vi "RFmxSpecAn CHP (Analysis Only) with Recommended Settings -Out of the Box.vi"() -> ()   [LabVIEW 2017]
doc: "This example illustrates how to use NI-RFmx in hardware agnostic mode to perform measurements on user provided IQ or Spectrum waveform. The example uses NI-RFSA driver API to acquire waveform from NI RF Signal Analyzer and perform an ACP measurement. The NI-RFSA acquisition settings are read from NI-RFmx session after Commit VI call. The NI-RFmx session is opened with Option String set as \"AnalysisOnly=1\"."
uses:
  <vilib>/Utility/error.llb/DialogType.ctl
  <instrlib>/niRFSA/niRFSA.llb/niRFSA Fetch IQ (1D Complex WDT NRec 1Chan).vi
  <vilib>/Analysis/1siggen.llb/Ramp Pattern by Delta.vi
  <vilib>/RFmx/SpecAn/mx/RFmxSpecAn.llb/RFmxSpecAn Analyze (IQ).vi
  <vilib>/RFmx/SpecAn/mx/RFmxSpecAn.llb/RFmxSpecAn CHP Fetch Measurement.vi
  <vilib>/Analysis/NI_AALBase.lvlib
  <vilib>/RFmx/SpecAn/mx/RFmxSpecAn.llb/RFmxSpecAn TXP Fetch Power Trace.vi
panel:
  out "Array":dbl[](array[numeric])
  out "XY Graph":cluster{"Ramp Pattern":dbl[], dbl[]}(graph)
  in  "Resource Name Test Signal Generation":refnum<k15>="RFSG" caption="resource name"
  in  "number of records":i64=10
  in  "Carrier Frequency (Hz)":dbl=4000000000.0 format="%#_6p"
  in  "Resource Name 2":refnum<k15>="RFSA" caption="Resource Name"
  in  "Reference Level (dBm)":dbl format="%.2f"
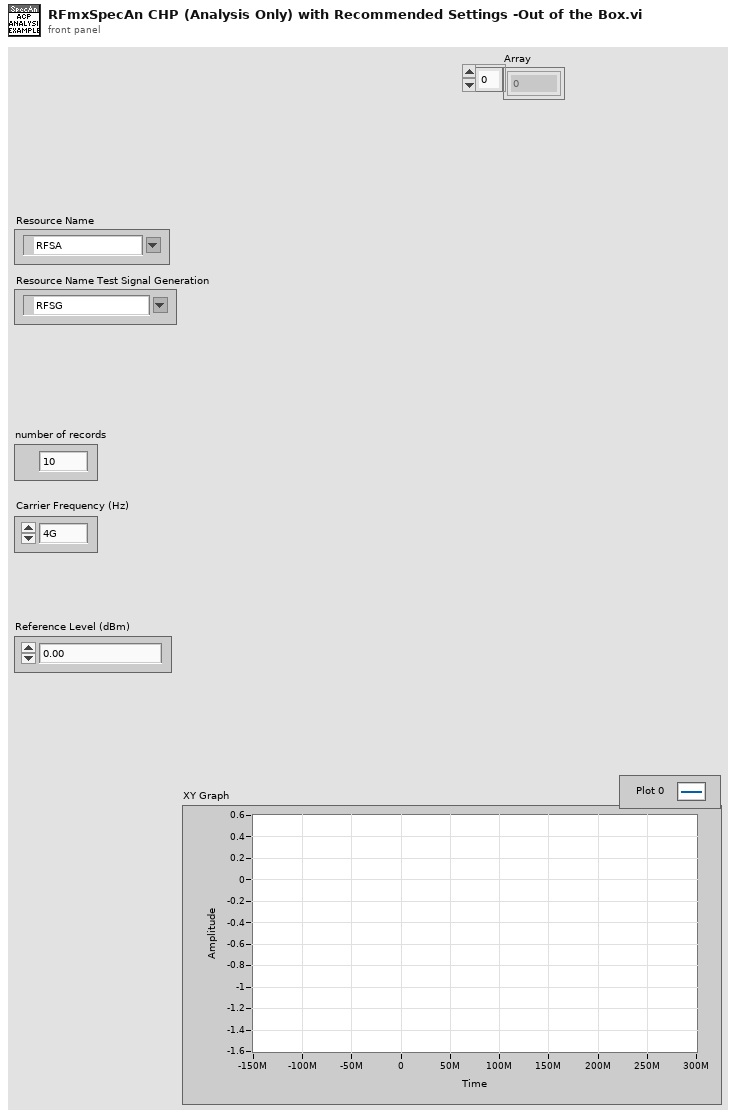
[diagram p1: front panel]
types:
  T1 = typedef "DialogType.ctl" = u16
  T2 = typedef "niRFmx Instrument Handle.ctl" = refnum<k21>
  T3 = enum16{"open", "open or create", "create or replace", "create", "open (read-only)"}
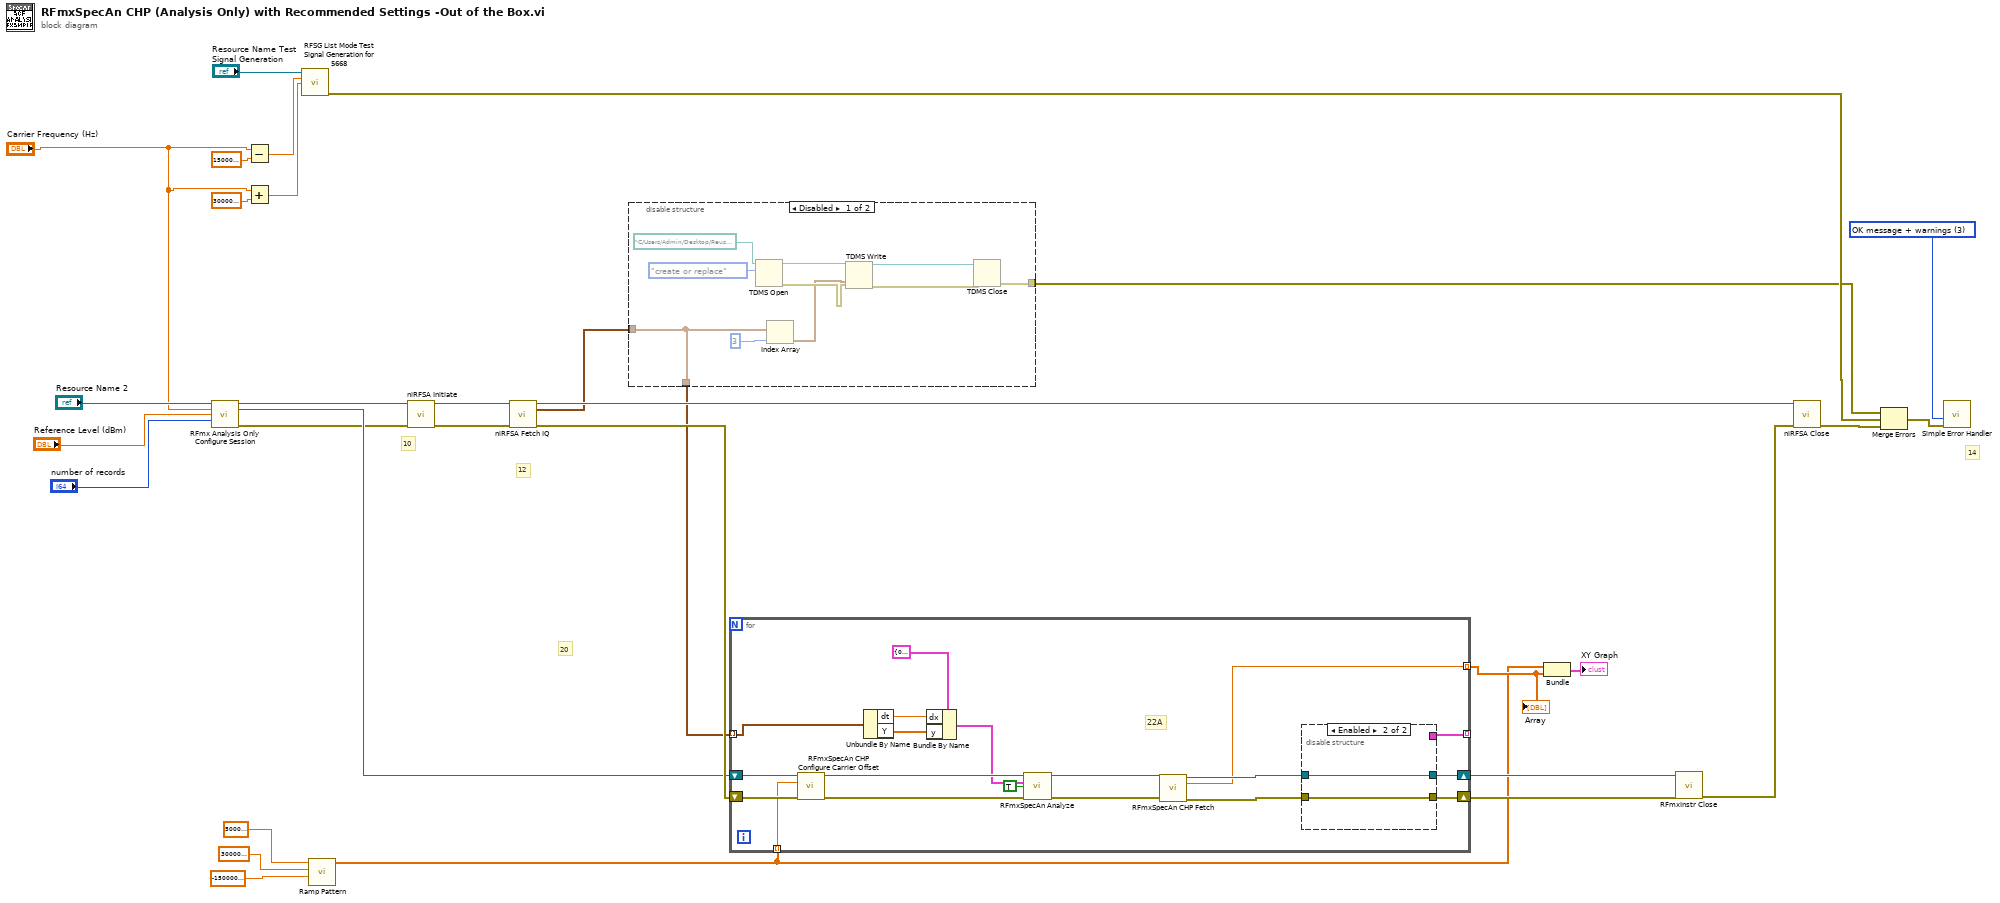
[diagram p0: block diagram]
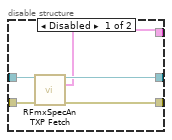
[diagram p3: hidden frame]
diagram:
  w31 = T1 3 items=["no dialog", "OK message", "continue or stop message", "OK message + warnings", "continue/stop + warnings"] ("type of dialog (OK msg:1)")
  # "12"
  # "10"
  # "14"
  # "20"
  n1 = call "RFmx Analysis Only Configure Session.vi"("IVI Refnum in"="Resource Name 2", "Carrier Frequency (Hz)"="Carrier Frequency (Hz)", "Reference Level (dBm)"="Reference Level (dBm)", "number of records"="number of records") -> ("RFSA Instrument Handle Out"=w28:refnum<k15>, "RFmx Instrument Handle Out"=w24:T2, "error out 2"=w16:errorcluster)  [unwired: 9 in]
  n2 = Subtract(x="Carrier Frequency (Hz)", y=150000000.0) -> (x-y=w13:dbl)
  n3 = Add(x="Carrier Frequency (Hz)", y=300000000.0) -> (x+y=w12:dbl)
  n4 = call "RFSG List Mode Test Signal Generation for 5668.vi"("Resource Name"="Resource Name Test Signal Generation", "Start Frequency"=w13, "End Frequency"=w12) -> ("error out"=w6:errorcluster)  [unwired: 11 in, 1 out]
  n5 = call-poly <vilib>:"Ramp Pattern.vi"("start"=-150000000.0, "end"=300000000.0, "delta"=50000000.0) -> ("Ramp Pattern"=w2:dbl[])  [unwired: 6 in, 2 out]
  n6 = call <instrlib>:"niRFSA Initiate.vi"("instrument handle"=w28, "error in"=w16) -> ("instrument handle out"=w23:refnum<k15>, "error out"=w22:errorcluster)  [unwired: 12 in]
  n7 = call-poly <instrlib>:"niRFSA Fetch IQ.vi"("instrument handle"=w23, "error in"=w22) -> ("instrument handle out"=w30:refnum<k15>, "data"=w8:waveform(cdb)[], "error out"=w27:errorcluster)  [unwired: 11 in]
  n8 = disable-structure shown="Disabled" {
    disable-tunnel: [w36 _] -> w5
    disable-tunnel: w8 -> [w33 w43]
    disable-tunnel: [w33 w43] -> w7
    frame Disabled {
      n9 = TDMS Open(10:T3."create or replace" ("operation (0:open)"), 11:path "C:/Users/Admin/Desktop/Reuse/Scanning Speed PXIe 5668/Data8G.tdms.txt" ("file path")) -> (0:w40:errorcluster, 3:w39:refnum<k34>)  [unwired: 5 in]
      n10 = Index Array(array=w33, index=3) -> (element=w34:waveform(cdb))
      n11 = TDMS Write(0:w39, 9:w34, 11:w40) -> (4:w37:refnum<k34>, 15:w38:errorcluster)  [unwired: 3 in, 2 out]
      n12 = TDMS Close(8:w38, 11:w37) -> (0:w36:errorcluster)  [unwired: 1 out]
    }
    frame Enabled {
    }
  }
  n13 = for {
    shift-right: [w60] -> w25
    shift-left: w27 -> [w62]
    shift-right: [w61] -> w26
    shift-left: w24 -> [w49]
    tunnel: [w50] -> w3 mode=indexing
    tunnel: w7 -> [w48] mode=indexing
    tunnel: [w57] -> _ mode=indexing
    tunnel: w2 -> [w51] mode=indexing
    # "22A"
    n14 = call <vilib>:"RFmxSpecAn CHP Configure Carrier Offset.vi"("Instrument Handle In"=w49, "Carrier Frequency (Hz)"=w51, "error in (no error)"=w62) -> ("Instrument Handle Out"=w52:refnum<k21>, "error out"=w53:errorcluster)  [unwired: 11 in]
    n15 = Unbundle By Name(w48) -> ("dt"=w46:dbl, "Y"=w45:cdb[])
    n16 = Bundle By Name(cluster=cluster{"x0":dbl, "dx":dbl, "y":csg[]} {"x0"=0.0, "dx"=0.0, "y"=[]} ("IQ"), "dx"=w46, "y"=w45) -> (w44:cluster{"x0":dbl, "dx":dbl, "y":csg[]})
    n17 = call-poly <vilib>:"RFmxSpecAn Analyze.vi"("Instrument Handle In"=w52, "IQ"=w44, "Reset?"=TRUE, "error in (no error)"=w53) -> ("Instrument Handle Out"=w56:refnum<k21>, "error out"=w55:errorcluster)  [unwired: 8 in, 2 out]
    n18 = call-poly <vilib>:"RFmxSpecAn CHP Fetch.vi"("Instrument Handle In"=w56, "error in (no error)"=w55) -> ("Instrument Handle Out"=w54:refnum<k21>, "Absolute Power (dBm)"=w50:dbl, "error out"=w58:errorcluster)  [unwired: 8 in, 3 out]
    n19 = disable-structure shown="Enabled" {
      disable-tunnel: [w67 w69] -> w61
      disable-tunnel: [w66 w68] -> w60
      disable-tunnel: w58 -> [w65 w68]
      disable-tunnel: [w64 _] -> w57
      disable-tunnel: w54 -> [w63 w69]
      frame Disabled {
        n20 = call-poly <vilib>:"RFmxSpecAn TXP Fetch.vi"("Instrument Handle In"=w63, "error in (no error)"=w65) -> ("Instrument Handle Out"=w67:refnum<k21>, "Power (dBm)"=w64:cluster{"x0":dbl, "dx":dbl, "y":sgl[]}, "error out"=w66:errorcluster)  [unwired: 11 in]
      }
      frame Enabled {
      }
    }
  }
  "Array" <- w3
  n21 = Bundle("Ramp Pattern"=w2, w3) -> (→"XY Graph":cluster{"Ramp Pattern":dbl[], dbl[]})  [unwired: 1 in]
  n22 = call <vilib>:"RFmxInstr Close.vi"("Instrument Handle In"=w26, "error in (no error)"=w25) -> ("error out"=w32:errorcluster)  [unwired: 13 in]
  n23 = call <instrlib>:"niRFSA Close.vi"("instrument handle"=w30, "error in"=w32) -> ("error out"=w10:errorcluster)  [unwired: 13 in]
  n24 = Merge Errors(w5, w6, w10) -> (w9:errorcluster)
  n25 = call <vilib>:"Simple Error Handler.vi"("type of dialog (OK msg:1)"=w31, "error in (no error)"=w9) -> ()  [unwired: 3 in, 5 out]
